vi "LV1_4zecimal.vi"() -> ()   [LabVIEW 2016]
uses:
  <vilib>/Instr/_visa.llb/VISA Configure Serial Port (Instr).vi
panel:
  out "Meter":dbl(knob) scale=0.0..4100.0
  out "Tank":dbl(slide) scale=0.0..4100.0
  in  "offset":i32
  out "String":string
  out "Waveform Chart":i32(graph)
  in  "VISA resource name":refnum<visa-resource-name>
  in  "stop":bool
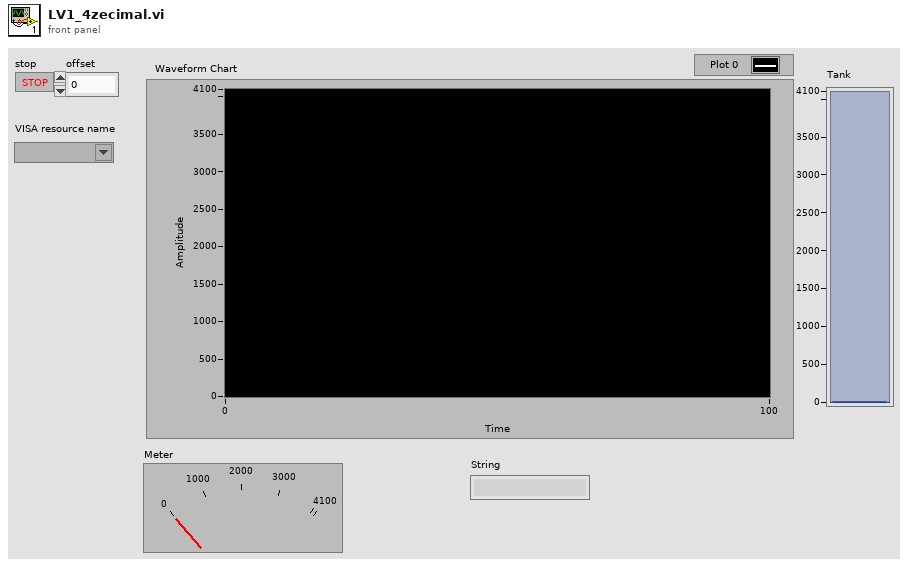
[diagram p1: front panel]
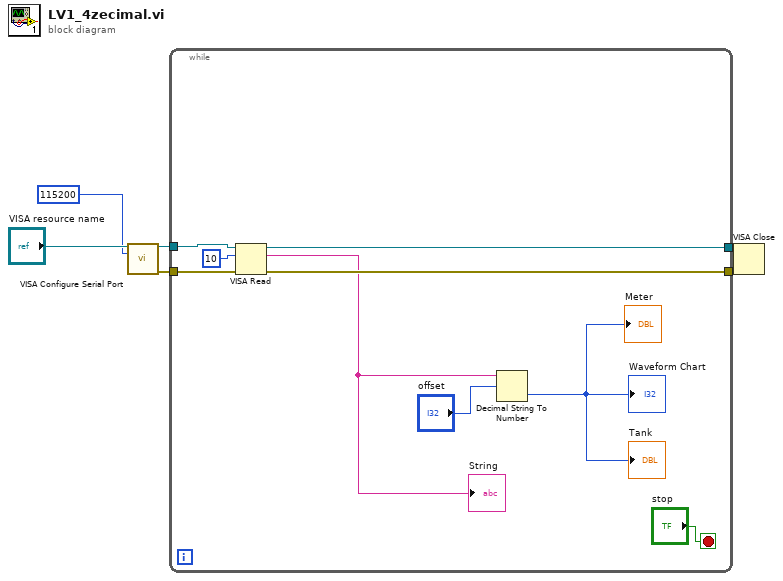
[diagram p0: block diagram]
diagram:
  n1 = call-poly "VISA Configure Serial Port"("VISA resource name"="VISA resource name", "baud rate (9600)"=u32 115200) -> ("VISA resource name out"=w6:refnum<visa-resource-name>, "error out"=w4:errorcluster)  [unwired: 12 in]
  n2 = while {
    tunnel: w6 -> [w14]
    tunnel: [w7] -> w5
    tunnel: w4 -> [w13]
    tunnel: [w12] -> w3
    stop <- "stop" stop-if-true
    n3 = VISA Read(VISA resource name=w14, byte count=u32 10, error in (no error)=w13) -> (VISA resource name out=w7:refnum<visa-resource-name>, read buffer=w9:string, error out=w12:errorcluster)  [unwired: 1 out]
    "String" <- w9
    n4 = Decimal String To Number(string=w9, offset="offset") -> (number=→"Waveform Chart" →"Tank" →"Meter":i32)  [unwired: 1 in, 1 out]
  }
  n5 = VISA Close(VISA resource name=w5, error in (no error)=w3) -> ()  [unwired: 1 out]
